vi "Get SPI Engine Commands 64-bit.vi"(6 "Ready for Output":bool, 8 "error in":errorcluster, 11 "SPI Engine Resources":T1={"To SPI Engine Data FIFO"="DLU To SPI Engine Data FIFO", "From SPI Engine Data FIFO"="SPI Engine to DLU Data FIFO", "Data to SPI Engine Cache Register"="Data to SPI Engine (Cache)", "SPI Transaction Settings Cache Register"="SPI PHY Settings to SPI Engine (Cache)"}) -> (0 "error out":errorcluster, 1 "Output Valid":bool, 2 "SPI Transaction Packet":T2 {"SPI Settings"."SPI Physical Settings"."Direction Change Bit" max=64 step=1; "SPI Settings"."SPI Physical Settings"."Transfer Length (bits)" min=1 max=64 step=1}, 3 "SPI Engine Resources":T1={"To SPI Engine Data FIFO"="DLU To SPI Engine Data FIFO", "From SPI Engine Data FIFO"="SPI Engine to DLU Data FIFO", "Data to SPI Engine Cache Register"="Data to SPI Engine (Cache)", "SPI Transaction Settings Cache Register"="SPI PHY Settings to SPI Engine (Cache)"}, 5 "Start Strobe":bool)   [LabVIEW 2015, in "SPI API.lvlib"]
uses:
  SPI API.lvlib
  Controls/SPI API Transaction Packet 64-bit.ctl
  Controls/SPI API Data 64-bit.ctl
  Controls/SPI Transaction Settings.ctl
  <userlib>/_NI SPI IP/FPGA/Controllers/Public/Transfer Settings.ctl
  Controls/SPI Engine Resources 64-bit.ctl
  Controls/SPI API Engine Receiver States.ctl
  SPI Engine.Get Commands.Read FIFO 64-bit.vi
  <userlib>/_NI SPI IP/FPGA/Controllers/NI SPI IP FPGA.lvlib
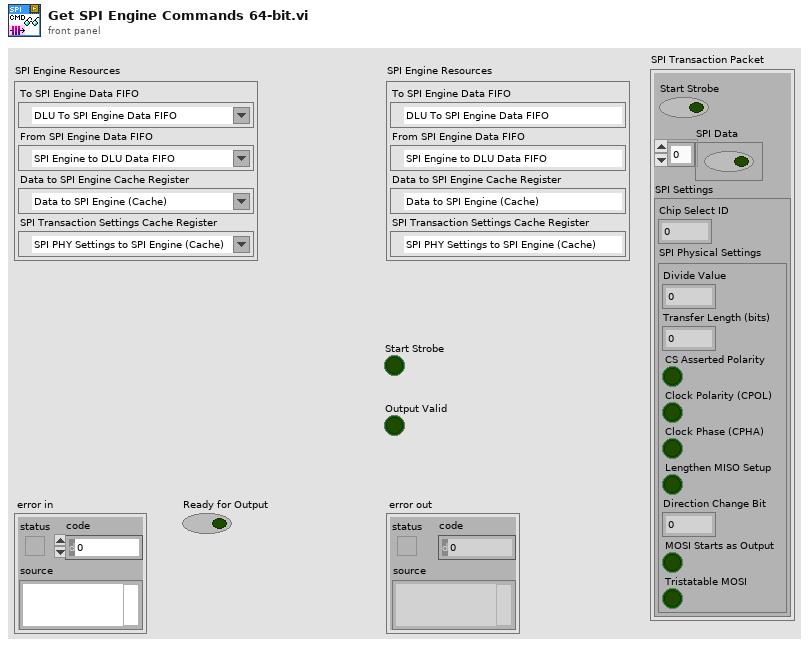
[diagram p1: front panel]
types:
  T1 = typedef "SPI API.lvlib/SPI Engine Resources 64-bit.ctl" = cluster{"To SPI Engine Data FIFO":refnum<k21>, "From SPI Engine Data FIFO":refnum<k21>, "Data to SPI Engine Cache Register":refnum<k21>, "SPI Transaction Settings Cache Register":refnum<k21>}
  T2 = typedef "SPI API.lvlib/SPI API Transaction Packet 64-bit.ctl" = cluster{"Start Strobe":bool, "SPI Data":T3, "SPI Settings":T4}
  T3 = typedef "SPI API.lvlib/SPI API Data 64-bit.ctl" = bool[]
  T4 = typedef "SPI API.lvlib/SPI Transaction Settings.ctl" = cluster{"Chip Select ID":u8, "SPI Physical Settings":T5}
  T5 = typedef "NI SPI IP FPGA.lvlib/Transfer Settings.ctl" = cluster{"Divide Value":u8, "Transfer Length (bits)":u8, "CS Asserted Polarity":bool, "Clock Polarity (CPOL)":bool, "Clock Phase (CPHA)":bool, "Lengthen MISO Setup":bool, "Direction Change Bit":u8, "MOSI Starts as Output":bool, "Tristatable MOSI":bool}
  T6 = typedef "SPI API.lvlib/SPI API Engine Receiver States.ctl" = enum16{"Wait for Start Command", "Deassert Start Probe"}
  T7 = typedef "SPI API.lvlib/SPI API Transmit Data 64-bit.ctl" = cluster{"SPI Data":T3, "SPI Settings":T4}
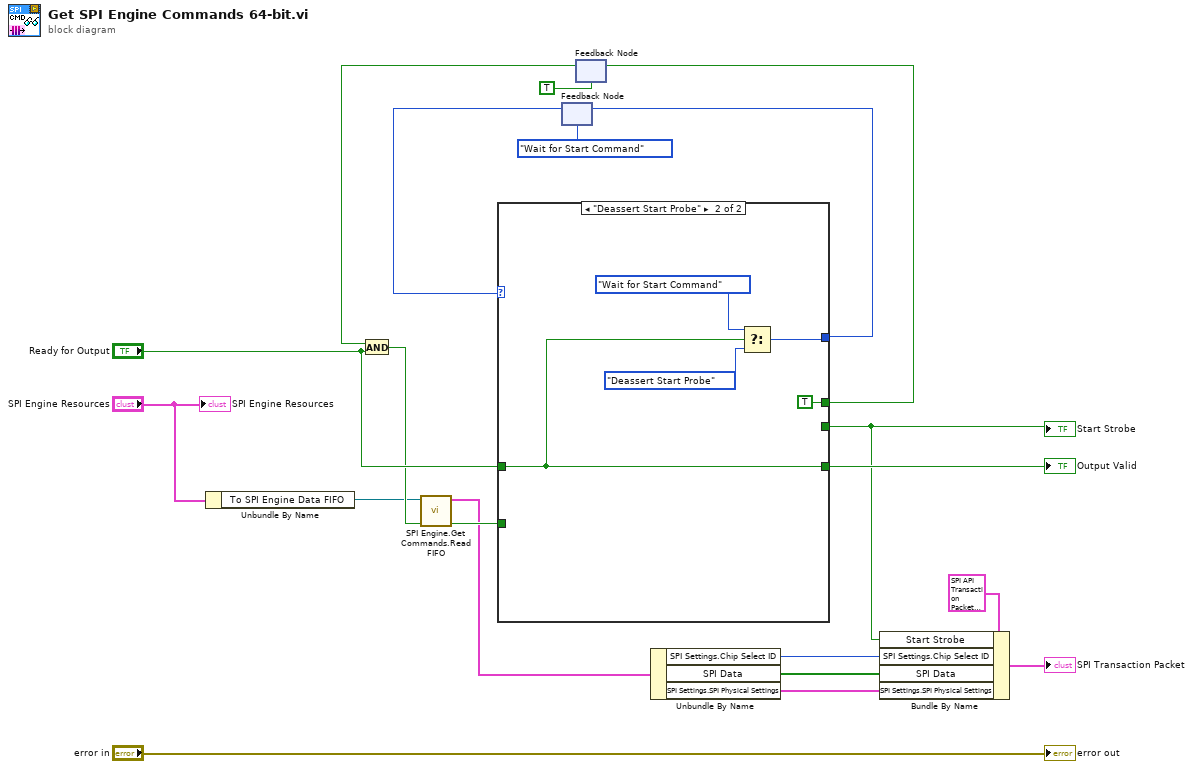
[diagram p0: block diagram]
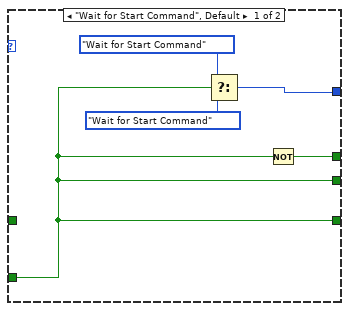
[diagram p2: hidden frame]
diagram:
  n1 = Unbundle By Name("SPI Engine Resources") -> ("To SPI Engine Data FIFO"=w1:refnum<k21>)
  n2 = feedback #1(SPI_API_Engine_Receiver_States."Wait for Start Command") -> (w19:T6)
  n3 = feedback #2(TRUE) -> (w16:bool)
  n4 = And(x=w16, y="Ready for Output") -> (x .and. y?=w4:bool)
  n5 = call-poly "SPI Engine.Get Commands.Read FIFO.vi"("Get New Data"=w4, "To SPI Engine Data FIFO"=w1) -> ("Output Valid"=w3:bool, "SPI Transaction Packet"=w2:T7)  [unwired: 8 in]
  n6 = case shown="\"Deassert Start Probe\"" w19 {
    tunnel: [w23 w26] -> w18
    tunnel: [w22 TRUE] -> w17
    tunnel: w3 -> [w21 _]
    tunnel: [w21 _] -> w6
    tunnel: [w21 w28] -> w14
    tunnel: "Ready for Output" -> [_ w28]
    frame "Wait for Start Command", Default {
      n7 = Select(t=SPI_API_Engine_Receiver_States."Wait for Start Command", s=w21, f=SPI_API_Engine_Receiver_States."Wait for Start Command") -> (s? t:f=w23:T6)
      n8 = Not(x=w21) -> (.not. x?=w22:bool)
    }
    frame "Deassert Start Probe" {
      n9 = Select(t=SPI_API_Engine_Receiver_States."Wait for Start Command", s=w28, f=SPI_API_Engine_Receiver_States."Deassert Start Probe") -> (s? t:f=w26:T6)
    }
  }
  "Start Strobe" <- w6
  "Output Valid" <- w14
  n10 = feedback-in #1(w18) -> ()
  n11 = feedback-in #2(w17) -> ()
  n12 = Unbundle By Name(w2) -> ("SPI Settings.Chip Select ID"=w11:u8, "SPI Data"=w10:T3, "SPI Settings.SPI Physical Settings"=w9:T5)
  n13 = Bundle By Name(cluster=T2 {"Start Strobe"=FALSE, "SPI Data"=[FALSE, FALSE, FALSE, FALSE, FALSE, FALSE, FALSE, FALSE, FALSE, FALSE, FALSE, FALSE, FALSE, FALSE, FALSE, FALSE, FALSE, FALSE, FALSE, FALSE, FALSE, FALSE, FALSE, FALSE, FALSE, FALSE, FALSE, FALSE, FALSE, FALSE, FALSE, FALSE, FALSE, FALSE, FALSE, FALSE, FALSE, FALSE, FALSE, FALSE, FALSE, FALSE, FALSE, FALSE, FALSE, FALSE, FALSE, FALSE, FALSE, FALSE, FALSE, FALSE, FALSE, FALSE, FALSE, FALSE, FALSE, FALSE, FALSE, FALSE, FALSE, FALSE, FALSE, FALSE], "SPI Settings"={"Chip Select ID"=0, "SPI Physical Settings"={"Divide Value"=0, "Transfer Length (bits)"=0, "CS Asserted Polarity"=FALSE, "Clock Polarity (CPOL)"=FALSE, "Clock Phase (CPHA)"=FALSE, "Lengthen MISO Setup"=FALSE, "Direction Change Bit"=0, "MOSI Starts as Output"=FALSE, "Tristatable MOSI"=FALSE}}} ("SPI Transaction Packet"), "Start Strobe"=w6, "SPI Settings.Chip Select ID"=w11, "SPI Data"=w10, "SPI Settings.SPI Physical Settings"=w9) -> (→"SPI Transaction Packet":T2)
  "error out" <- "error in"
  "SPI Engine Resources" <- "SPI Engine Resources"
